vi "[FGV]MaskROIDataEntry.vi"(0 "ROI":T2(array[cluster]), 1 "[FGV]MaskROIList_Action":T3, 5 "ROIIn":T1, 7 "ROINameIn":string[](array[string]), 9 "Replace index":i32, 11 "error in (no error)":errorcluster) -> (4 "ROIArrayOut":T2(array[cluster]), 6 "ROINameOut":string[](array[string]), 15 "error out":errorcluster)   [LabVIEW 2019]
uses:
  Controls/MaskROIList_Action.ctl
panel:
  in  "ROIName":string[](array[string])
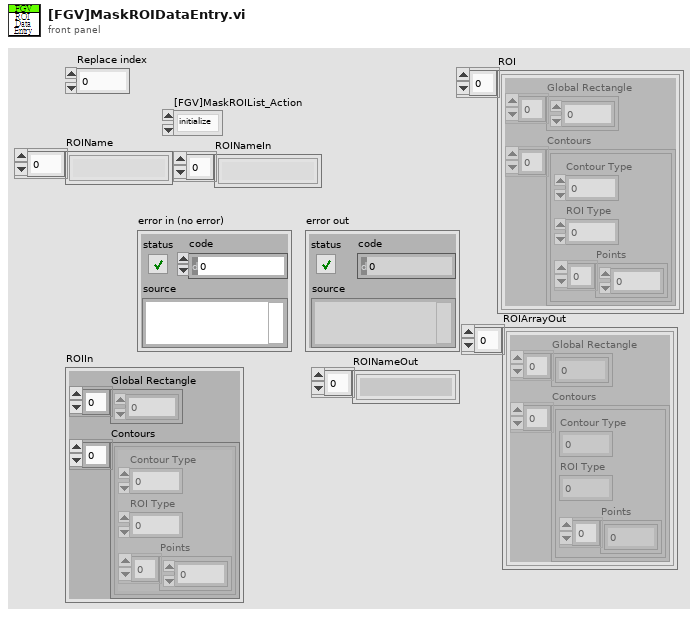
[diagram p1: front panel]
types:
  T1 = cluster{"Global Rectangle":i32[], "Contours":cluster{"Contour Type":u32, "ROI Type":u32, "Points":i32[]}[]}
  T2 = cluster{"Global Rectangle":i32[], "Contours":cluster{"Contour Type":u32, "ROI Type":u32, "Points":i32[]}[]}[]
  T3 = typedef "MaskROIList_Action.ctl" = enum16{"initialize", "SaveAll", "ReadAll", "Append", "Replace", "DeleteIndex"}
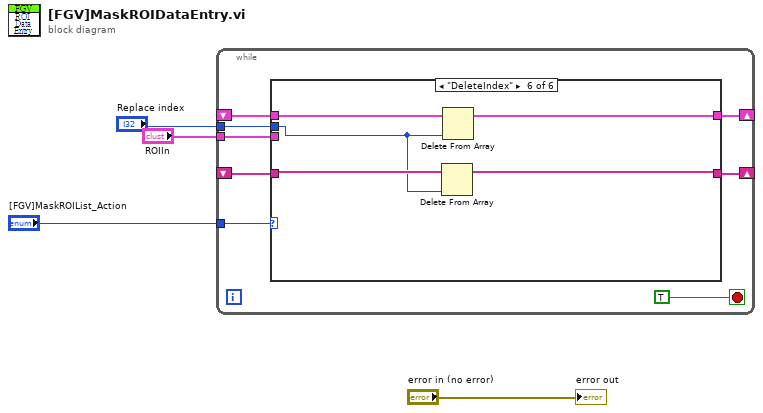
[diagram p0: block diagram]
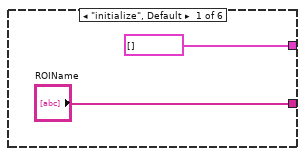
[diagram p2: hidden frame]
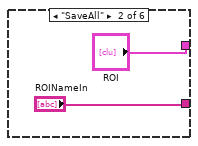
[diagram p3: hidden frame]
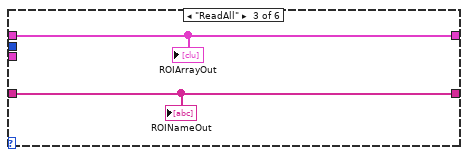
[diagram p4: hidden frame]
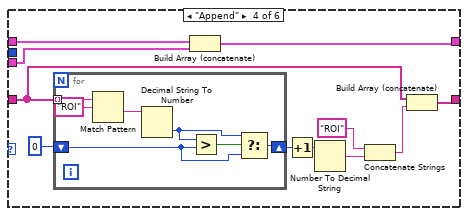
[diagram p5: hidden frame]
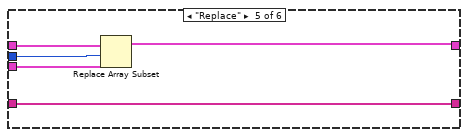
[diagram p6: hidden frame]
diagram:
  n1 = while {
    tunnel: "[FGV]MaskROIList_Action" -> [w11]
    shift-right: [w10] -> _
    shift-left: _ -> [w9]
    shift-right: [w8] -> _
    shift-left: _ -> [w7]
    tunnel: "ROIIn" -> [w6]
    tunnel: "Replace index" -> [w5]
    stop <- TRUE stop-if-true
    n2 = case shown="\"DeleteIndex\"" w11 {
      tunnel: [T2 [] ("ROI") "ROI" w18 w28 w39 w43] -> w10
      tunnel: w9 -> [_ _ w18 w29 w40 w46]
      tunnel: ["ROIName" "ROINameIn" w17 w21 w41 w42] -> w8
      tunnel: w7 -> [_ _ w17 w23 w41 w45]
      tunnel: w6 -> [_ _ _ w19 w38 _]
      tunnel: w5 -> [_ _ _ _ w37 w44]
      frame "initialize", Default {
      }
      frame "SaveAll" {
      }
      frame "ReadAll" {
        "ROIArrayOut" <- w18
        "ROINameOut" <- w17
      }
      frame "Append" {
        n3 = for {
          tunnel: w23 -> [w36] mode=indexing
          shift-right: [w30] -> w26
          shift-left: 0 -> [w31]
          n4 = Match Pattern(string=w36, regular expression="ROI") -> (after substring=w34:string)  [unwired: 1 in, 3 out]
          n5 = Decimal String To Number(string=w34) -> (number=w32:i32)  [unwired: 2 in, 1 out]
          n6 = Greater?(x=w32, y=w31) -> (0:w33:bool)
          n7 = Select(t=w32, s=w33, f=w31) -> (s? t:f=w30:i32)
        }
        n8 = Build Array (concatenate)(w29, w19) -> (w28:T2)
        n9 = Increment(x=w26) -> (x+1=w20:i32)
        n10 = Number To Decimal String(number=w20) -> (decimal integer string=w25:string)  [unwired: 1 in]
        n11 = Concatenate Strings("ROI", w25) -> (w22:string)
        n12 = Build Array (concatenate)(w23, w22) -> (w21:string[])
      }
      frame "Replace" {
        n13 = Replace Array Subset(array=w40, new element=w38, index=w37) -> (w39:T2)
      }
      frame "DeleteIndex" {
        n14 = Delete From Array(array=w45, index=w44) -> (array with subset deleted=w42:string[])  [unwired: 1 in, 1 out]
        n15 = Delete From Array(array=w46, index=w44) -> (array with subset deleted=w43:T2)  [unwired: 1 in, 1 out]
      }
    }
  }
  "error out" <- "error in (no error)"
